vi "Start Sync.vi"(8 "error in (no error)":errorcluster, 11 "gRPC Server in":refnum<class "OOP Query Server.lvclass">) -> (0 "error out":errorcluster, 3 "gRPC Server out":refnum<class "OOP Query Server.lvclass">)   [LabVIEW 2019, in "OOP Query Server.lvlib" / "OOP Query Server.lvclass"]
uses:
  OOP Query Server.lvclass
  gRPC interface/Server API/typeDefs/grpcId.ctl
  OOP Query Server.lvclass/OOP Query Server.ctl
  RPC Messages/ServerEvent/ServerEvent_Data.ctl
  RPC Messages/InvokeResponse/InvokeResponse_Data.ctl
  RPC Messages/QueryResponse/QueryResponse_Data.ctl
  gRPC interface/gprc-lvsupport.lvlib
  OOP Server/Class/OOP Server.lvclass
  gRPC lvSupport/Server API/typeDefs/grpcId.ctl
  gRPC lvSupport/gprc-lvsupport.lvlib
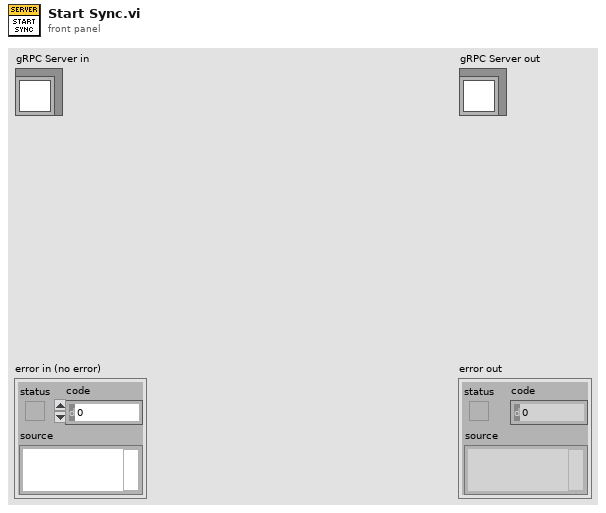
[diagram p1: front panel]
types:
  T1 = typedef "OOP Query Server.lvlib/OOP Query Server.lvclass/ServerEvent_Data.ctl" = cluster{"eventData":string, "serverId":i32, "status":i32}
  T2 = typedef "OOP Query Server.lvlib/OOP Query Server.lvclass/InvokeResponse_Data.ctl" = cluster{"status":i32}
  T3 = typedef "OOP Query Server.lvlib/OOP Query Server.lvclass/QueryResponse_Data.ctl" = cluster{"message":string, "status":i32}
  T4 = typedef "OOP Query Server.lvlib/gprc-lvsupport.lvlib/grpcId.ctl" = u64
  T5 = typedef "OOP Query Server.lvlib/OOP Query Server.lvclass/Server gRPC UEs.ctl" = cluster{"Invoke gRPC UE":refnum<user-event>, "Query gRPC UE":refnum<user-event>, "Register gRPC UE":refnum<user-event>}
  T6 = typedef "OOP Server.lvlib/OOP Server.lvclass/InvokeRequest_Data.ctl" = cluster{"command":string, "parameter":string}
  T7 = typedef "gprc-lvsupport.lvlib/grpcId.ctl" = u64
  T8 = typedef "OOP Query Server.lvlib/OOP Query Server.lvclass/QueryRequest_Data.ctl" = cluster{"query":string}
  T9 = typedef "OOP Query Server.lvlib/OOP Query Server.lvclass/RegistrationRequest_Data.ctl" = cluster{"eventName":string}
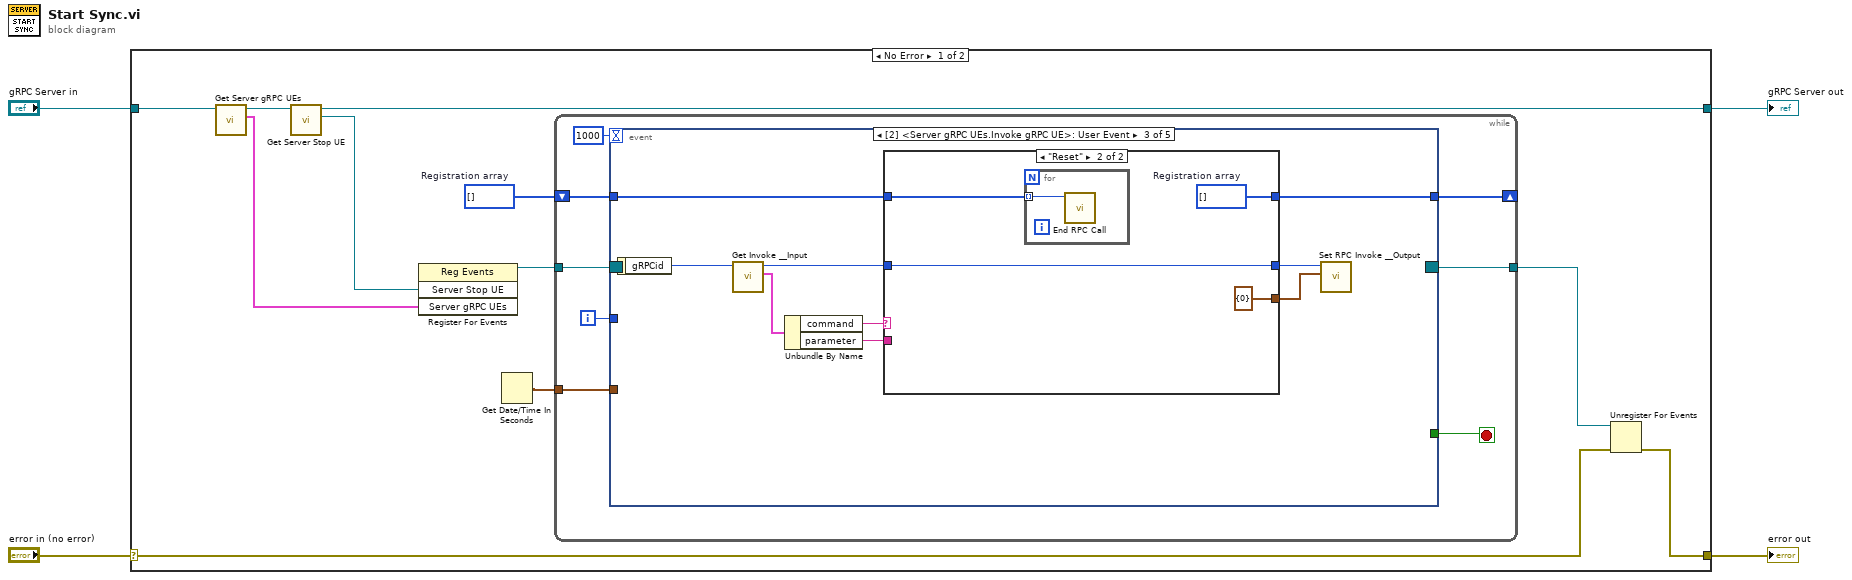
[diagram p0: block diagram]
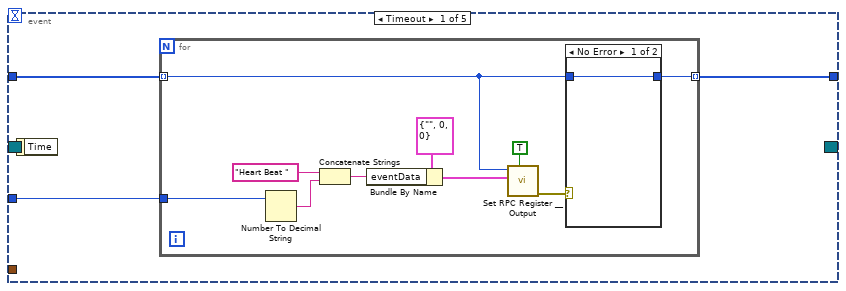
[diagram p2: hidden frame]
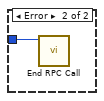
[diagram p3: hidden frame]
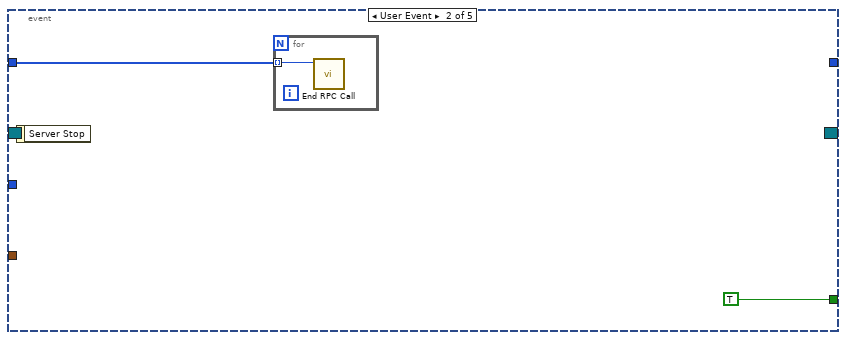
[diagram p4: hidden frame]
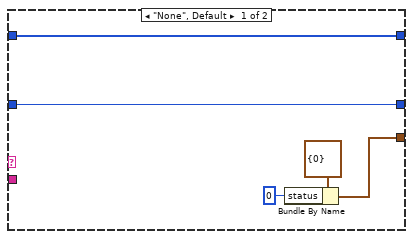
[diagram p5: hidden frame]
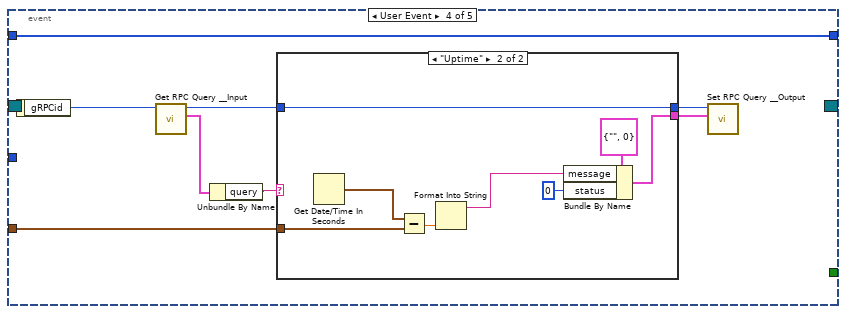
[diagram p6: hidden frame]
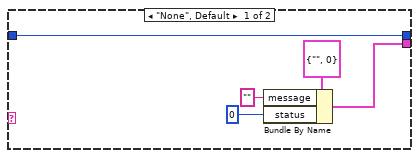
[diagram p7: hidden frame]
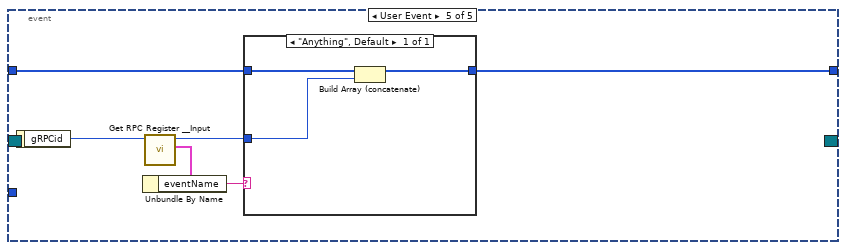
[diagram p8: hidden frame]
diagram:
  n1 = case shown="No Error" "error in (no error)" {
    selector: "error in (no error)" -> [w8 w92]
    tunnel: [w7 w92] -> w3
    tunnel: [w11 w91] -> w1
    tunnel: "gRPC Server in" -> [w15 w91]
    frame No Error {
      w6 = T4[] []  # Registration array
      n2 = call "Get Server gRPC UEs.vi"("OOP Server in"=w15) -> ("Server gRPC UEs"=w12:T5, "OOP Server out"=w14:refnum<class "OOP Query Server.lvclass">)  [unwired: 9 in]
      n3 = call "Get Server Stop UE.vi"("OOP Server in"=w14) -> ("Server Stop UE"=w13:refnum<user-event>, "OOP Server out"=w11:refnum<class "OOP Query Server.lvclass">)  [unwired: 9 in]
      n4 = register-events(w13, w12) -> (reference out=w10:refnum<event-registration>)  [unwired: 2 in, 1 out]
      n5 = Get Date/Time In Seconds() -> (seconds since 1Jan1904=w5:timestamp)
      n6 = while {
        tunnel: w10 -> [w23]
        tunnel: [w21] -> w9
        shift-right: [w18] -> _
        shift-left: w6 -> [w19]
        tunnel: w5 -> [w16]
        i -> [w17]
        stop <- w22 stop-if-true
        n7 = event "RPC Methods Event Structure" shown="[2] <Server gRPC UEs.Invoke gRPC UE>: User Event" {
          selector: w23 -> [_ _ _ _ _]
          dyn-events: [_ _ _ _ _] -> w21
          timeout: 1000 -> [_ _ _ _ _]
          tunnel: [_ TRUE _ _ _] -> w22
          tunnel: w19 -> [w26 w39 w43 w61 w83]
          tunnel: [w25 _ w42 w61 w82] -> w18
          tunnel: w17 -> [w24 _ _ _ _]
          tunnel: w16 -> [_ _ _ w62 _]
          event Timeout {
            n8 = event-data() -> ()  [unwired: 1 in, 1 out]
            n9 = for {
              tunnel: w26 -> [w28] mode=indexing
              tunnel: w24 -> [w30]
              tunnel: [w27] -> w25 mode=indexing
              n10 = Number To Decimal String(number=w30) -> (decimal integer string=w34:string)  [unwired: 1 in]
              n11 = Concatenate Strings("Heart Beat " ("eventdata"), w34) -> (w32:string)
              n12 = Bundle By Name(cluster=T1 {"eventData"="", "serverId"=0, "status"=0} ("Message Data"), "eventData"=w32) -> (w31:T1)
              n13 = call "Set RPC Register __Output.vi"("Streeming? (F)"=TRUE, "Message Data"=w31, "gRPCid in"=w28) -> ("error out"=w29:errorcluster)  [unwired: 8 in]
              n14 = case shown="No Error" w29 {
                tunnel: w28 -> [w37 w38]
                tunnel: [w37 _] -> w27
                frame No Error {
                }
                frame Error {
                  n15 = call "End RPC Call.vi"("gRPCid"=w38) -> ()  [unwired: 10 in, 1 out]
                }
              }
            }
          }
          event User Event {
            n16 = event-data() -> ()  [unwired: 1 in, 1 out]
            n17 = for {
              tunnel: w39 -> [w41] mode=indexing
              n18 = call "End RPC Call.vi"("gRPCid"=w41) -> ()  [unwired: 10 in, 1 out]
            }
          }
          event User Event {
            n19 = event-data() -> ("gRPCid"=w44:T4)  [unwired: 1 in]
            n20 = call "Get Invoke __Input.vi"("gRPCid"=w44) -> ("Message Data"=w50:T6, "gRPCid"=w47:T4)  [unwired: 8 in, 1 out]
            n21 = Unbundle By Name(w50) -> ("command"=w49:string, "parameter"=w48:string)
            n22 = case shown="\"Reset\"" w49 {
              tunnel: w48 -> [_ _]
              tunnel: w47 -> [w55 w58]
              tunnel: [w55 w58] -> w46
              tunnel: [w52 T2 {"status"=0} ("Message Data")] -> w45
              tunnel: w43 -> [w51 w59]
              tunnel: [w51 w56] -> w42
              frame "None", Default {
                n23 = Bundle By Name(cluster=T2 {"status"=0} ("Message Data"), "status"=0) -> (w52:T2)
              }
              frame "Reset" {
                w56 = T7[] []  # Registration array
                n24 = for {
                  tunnel: w59 -> [w60] mode=indexing
                  n25 = call "End RPC Call.vi"("gRPCid"=w60) -> ()  [unwired: 10 in, 1 out]
                }
              }
            }
            n26 = call "Set RPC Invoke __Output.vi"("Message Data"=w45, "gRPCid in"=w46) -> ()  [unwired: 9 in, 1 out]
          }
          event User Event {
            n27 = event-data() -> ("gRPCid"=w63:T4)  [unwired: 1 in]
            n28 = call "Get RPC Query __Input.vi"("gRPCid in"=w63) -> ("Message Data"=w68:T8, "gRPCid out"=w66:T4)  [unwired: 8 in, 1 out]
            n29 = Unbundle By Name(w68) -> ("query"=w67:string)
            n30 = case shown="\"Uptime\"" w67 {
              tunnel: w66 -> [w73 w81]
              tunnel: [w73 w81] -> w65
              tunnel: w62 -> [_ w77]
              tunnel: [w70 w74] -> w64
              frame "None", Default {
                n31 = Bundle By Name(cluster=T3 {"message"="", "status"=0} ("Message Data"), "message"="", "status"=0) -> (w70:T3)
              }
              frame "Uptime" {
                n32 = Get Date/Time In Seconds() -> (seconds since 1Jan1904=w79:timestamp)
                n33 = Subtract(x=w79, y=w77) -> (x-y=w78:dbl)
                n34 = Format Into String(w78) -> (resulting string=w76:string)  [unwired: 3 in, 1 out]
                n35 = Bundle By Name(cluster=T3 {"message"="", "status"=0} ("Message Data"), "message"=w76, "status"=0) -> (w74:T3)
              }
            }
            n36 = call "Set RPC Query __Output.vi"("Message Data"=w64, "gRPCid in"=w65) -> ()  [unwired: 9 in, 1 out]
          }
          event User Event {
            n37 = event-data() -> ("gRPCid"=w84:T4)  [unwired: 1 in]
            n38 = call "Get RPC Register __Input.vi"("gRPCid in"=w84) -> ("Message Data"=w87:T9, "gRPCid out"=w85:T4)  [unwired: 8 in, 1 out]
            n39 = Unbundle By Name(w87) -> ("eventName"=w86:string)
            n40 = case shown="\"Anything\", Default" w86 {
              tunnel: w85 -> [w90]
              tunnel: [w89] -> w82
              tunnel: w83 -> [w88]
              frame "Anything", Default {
                n41 = Build Array (concatenate)(w88, w90) -> (w89:T4[])
              }
            }
          }
        }
      }
      n42 = Unregister For Events(event registration refnum=w9, error in=w8) -> (error out=w7:errorcluster)
    }
    frame Error {
    }
  }
  "error out" <- w3
  "gRPC Server out" <- w1
